vi "Display Position.vi"() -> ()   [LabVIEW 2020]
panel:
  out "XY Graph":cluster{i32[], i32[]}(graph)
  in  "Table Control":string[][](table)
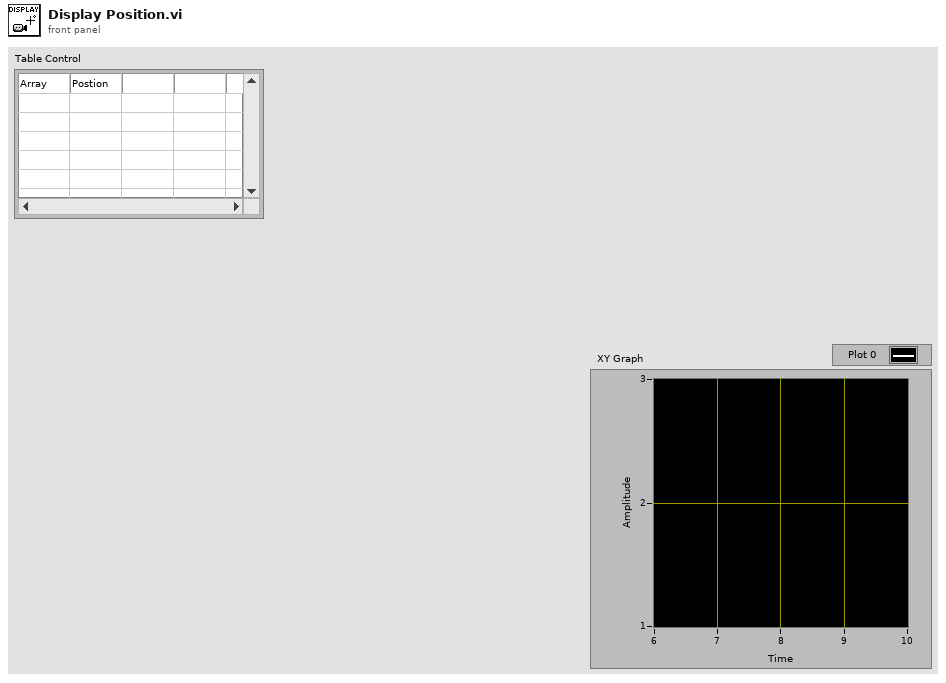
[diagram p1: front panel]
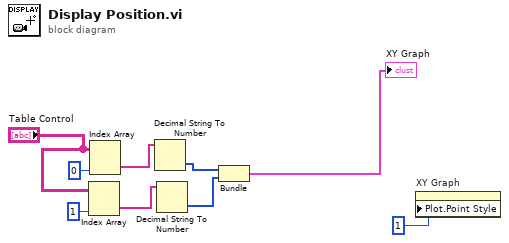
[diagram p0: block diagram]
diagram:
  n1 = Index Array(array="Table Control", index (col)=1) -> (element=w5:string[])  [unwired: 1 in]
  n2 = Index Array(array="Table Control", index (col)=0 ("disabled index (col)")) -> (element=w6:string[])  [unwired: 1 in]
  n3 = Decimal String To Number(string=w6) -> (number=w4:i32[])  [unwired: 2 in, 1 out]
  n4 = Decimal String To Number(string=w5) -> (number=w3:i32[])  [unwired: 2 in, 1 out]
  n5 = Bundle(w4, w3) -> (→"XY Graph":cluster{i32[], i32[]})  [unwired: 1 in]
  n6 = property on="XY Graph" class="XYGraph (strict)"("Plot.Point Style"=u8 1) -> ()  [unwired: 2 in, 2 out]
